vi "incrementActiveBridge.vi"(8 "error in (no error)":errorcluster, 11 "Model in":refnum<class "Model.lvclass">) -> (0 "error out":errorcluster, 3 "Model out":refnum<class "Model.lvclass">)   [LabVIEW 2013, in "Model.lvclass"]
uses:
  Model.lvclass
  Model.lvclass/Model.ctl
  ApplicationElements/Log/TestDataLog/TestDataLog.lvclass/TestDataLog.ctl
  UserEvents/UserEvents.lvclass/UserEvents.ctl
  ApplicationElements/TestMonitor/TestMonitor.lvclass/TestMonitor.ctl
  ApplicationElements/TestMonitor/TestMonitor.lvclass
  UserEvents/UserEvents.lvclass
  ApplicationElements/Log/TestDataLog/TestDataLog.lvclass
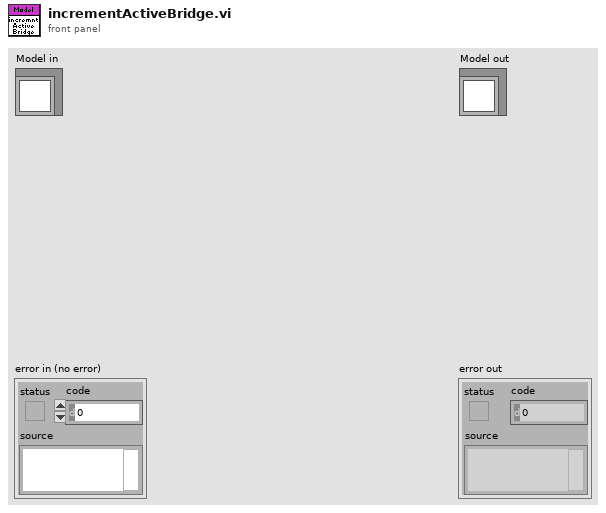
[diagram p1: front panel]
types:
  T1 = typedef "TestParameters.ctl" = cluster{"Number of cycles for complete test":u32, "Cycle profile":T2, "PGA Gain Coefficients":u8[], "Temperature Transition Wait Time":dbl[unit], "Temperature Settled StDev":dbl[unit], "Temperature Settling Sample Size":u16, "Bridge Measurement Sample Size":u16}
  T2 = typedef "CycleProfileConfig.ctl" = cluster{"Temperature Setpoint":dbl[unit][], "Soak Time":dbl[unit][], "Gain Stabilization Time":dbl[unit][], "Pause After Step":dbl[unit][]}
  T3 = typedef "AITDTTypedefs.lvlib/PubDataEvents.ctl" = cluster{"State":refnum<user-event>, "ErrorCode":refnum<user-event>, "OutputData":refnum<user-event>, "InputData":refnum<user-event>, "TestStatus":refnum<user-event>, "LogPath":refnum<user-event>, "TemperatureSetpointRequest":refnum<user-event>, "TemperatureSettling":refnum<user-event>, "WaitTimeStatus":refnum<user-event>}
  T4 = typedef "AITDTTypedefs.lvlib/TestStatus.ctl" = cluster{"activeCycle":u32, "activeProfileStep":u32, "demandedCycles":u32, "demandedProfileSteps":u32, "temperatureSetpoint":dbl[unit], "pgaGainCoefficient":u16}
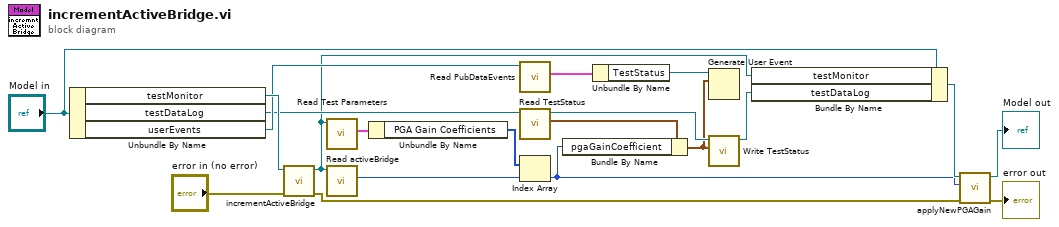
[diagram p0: block diagram]
diagram:
  n1 = Unbundle By Name("Model in") -> ("testMonitor"=w19:refnum<class "TestMonitor.lvclass">, "testDataLog"=w8:refnum<class "TestDataLog.lvclass">, "userEvents"=w9:refnum<class "UserEvents.lvclass">)
  n2 = call "incrementActiveBridge.vi"("error in (no error)"="error in (no error)", "TestMonitor in"=w19) -> ("error out"=w2:errorcluster, "TestMonitor out"=w7:refnum<class "TestMonitor.lvclass">)  [unwired: 8 in]
  n3 = call "Read Test Parameters.vi"("TestMonitor in"=w7) -> ("Test Parameters"=w12:T1)  [unwired: 9 in, 1 out]
  n4 = call "Read activeBridge.vi"("TestMonitor in"=w7) -> ("activeBridge"=w11:u32)  [unwired: 9 in, 1 out]
  n5 = Unbundle By Name(w12) -> ("PGA Gain Coefficients"=w10:u8[])
  n6 = call "Read PubDataEvents.vi"("UserEvents in"=w9) -> ("PubDataEvents"=w16:T3)  [unwired: 9 in, 1 out]
  n7 = call "Read TestStatus.vi"("Logger in"=w8) -> ("TestStatus"=w15:T4, "Logger out"=w17:refnum<class "TestDataLog.lvclass">)  [unwired: 9 in]
  n8 = Index Array(array=w10, index=w11) -> (element=w3:u8)
  n9 = Bundle By Name(cluster=w15, "pgaGainCoefficient"=w3) -> (w14:T4)
  n10 = Unbundle By Name(w16) -> ("TestStatus"=w13:refnum<user-event>)
  n11 = Generate User Event(user event=w13, event data cluster=w14) -> ()  [unwired: 2 in, 2 out]
  n12 = call "Write TestStatus.vi"("TestStatus"=w14, "Logger in"=w17) -> ("Logger out"=w6:refnum<class "TestDataLog.lvclass">)  [unwired: 9 in]
  n13 = Bundle By Name(cluster="Model in", "testMonitor"=w7, "testDataLog"=w6) -> (w5:refnum<class "Model.lvclass">)
  n14 = call "applyNewPGAGain.vi"("error in (no error)"=w2, "Preamplifier Gain"=w3, "Model in"=w5) -> ("error out"=→"error out":errorcluster, "Model out"=→"Model out":refnum<class "Model.lvclass">)  [unwired: 7 in]
